vi "initStorageFile.vi"   [LabVIEW 2010]
uses:
  AmmeterGlobalCostants.vi
types:
  T1 = enum16{"open", "replace", "create", "open or create", "replace or create", "replace or create with confirmation"}
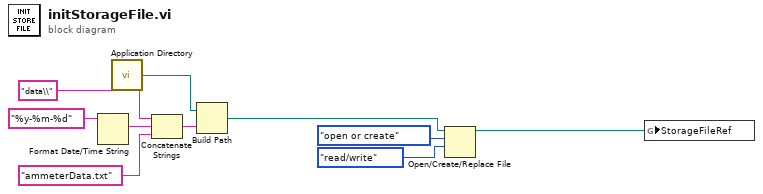
[diagram p0: block diagram]
diagram:
  n1 = Format Date/Time String(time format string (%c)="%y-%m-%d") -> (date/time string=w5:string)  [unwired: 2 in]
  n2 = call <vilib>:"Application Directory.vi"() -> ("Application Directory"=w10:path)
  n3 = Concatenate Strings("data\\" ("string"), w5, "ammeterData.txt" ("time format string (%c)")) -> (w3:string)
  n4 = Build Path(base path=w10, name or relative path=w3) -> (appended path=w7:path)
  n5 = Open/Create/Replace File(file path (use dialog)=w7, operation (0:open)=T1."open or create" ("操作(0:open)"), access (0:read/write)=enum16{"read/write", "read-only", "write-only"}."read/write" ("权限(0:read/write)")) -> (refnum out=w1:refnum<file>)  [unwired: 3 in, 2 out]
  n6 = global write "AmmeterGlobalCostants.vi" "StorageFileRef"(w1) -> ()
